vi "Build Flash Command.vi"(8 "error in":errorcluster, 11 "MPLab in":refnum<class "MPLab.lvclass">) -> (0 "error out":errorcluster, 3 "MPLab out":refnum<class "MPLab.lvclass">)   [LabVIEW 2018, in "MPLab.lvlib" / "MPLab.lvclass"]
uses:
  MPLab.lvclass
  Custom Controls/Command Line Options.ctl
  MPLab.lvclass/MPLab.ctl
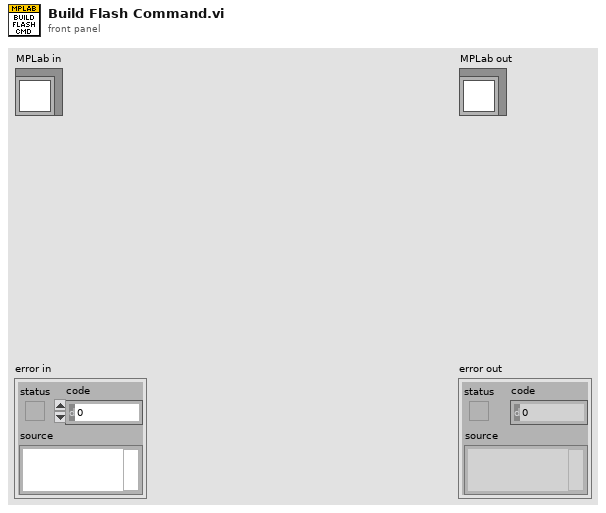
[diagram p1: front panel]
types:
  T1 = typedef "MPLab.lvlib/MPLab.lvclass/Command Line Options.ctl" = enum16{"Blank Check Device", "Erase Flash Device", "Hex File", "Display Device ID", "Display File Checksum", "Low Voltage Programming", "Memory Region", "Part", "Tool", "Verify Device"}
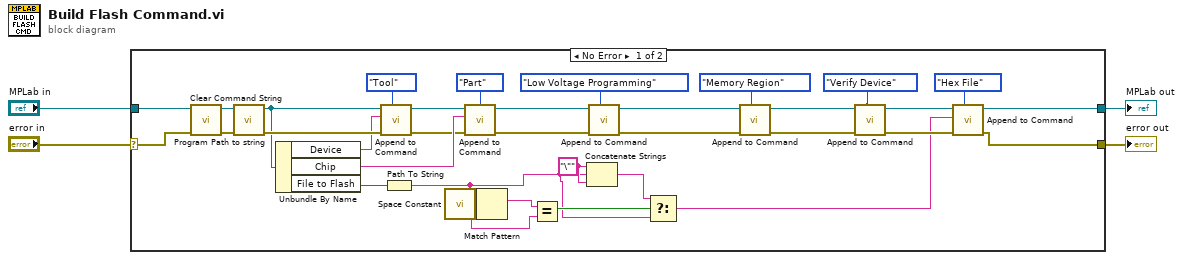
[diagram p0: block diagram]
diagram:
  n1 = case shown="No Error" "error in" {
    selector: "error in" -> [w36 w40]
    tunnel: [w12 w40] -> w3
    tunnel: [w13 w39] -> w1
    tunnel: "MPLab in" -> [w38 w39]
    frame No Error {
      w8 = "\"" ("string")
      n2 = call "Clear Command String.vi"("error in (no error)"=w36, "MPLab in"=w38) -> ("error out"=w35:errorcluster, "MPLab out"=w37:refnum<class "MPLab.lvclass">)  [unwired: 8 in]
      n3 = call "Program Path to string.vi"("error in"=w35, "MPLab in"=w37) -> ("error out"=w34:errorcluster, "MPLab out"=w33:refnum<class "MPLab.lvclass">)  [unwired: 8 in]
      n4 = Unbundle By Name(w33) -> ("Device"=w32:string, "Chip"=w29:string, "File to Flash"=w22:path)
      n5 = call "Append to Command.vi"("Command Line Options"=Command_Line_Options."Tool", "error in (no error)"=w34, "Parameter"=w32, "MPLab in"=w33) -> ("error out"=w23:errorcluster, "MPLab out"=w24:refnum<class "MPLab.lvclass">)  [unwired: 6 in]
      n6 = Path To String(path=w22) -> (string=w6:string)
      n7 = call <vilib>:"Space Constant.vi"() -> ("String"=w10:string)
      n8 = call "Append to Command.vi"("Command Line Options"=Command_Line_Options."Part", "error in (no error)"=w23, "Parameter"=w29, "MPLab in"=w24) -> ("error out"=w20:errorcluster, "MPLab out"=w21:refnum<class "MPLab.lvclass">)  [unwired: 6 in]
      n9 = Match Pattern(string=w6, regular expression=w10) -> (match substring=w11:string)  [unwired: 1 in, 3 out]
      n10 = Equal?(x=w11, y=w10) -> (x = y?=w9:bool)
      n11 = Concatenate Strings(w8, w6, w8) -> (w7:string)
      n12 = call "Append to Command.vi"("Command Line Options"=Command_Line_Options."Low Voltage Programming", "error in (no error)"=w20, "MPLab in"=w21) -> ("error out"=w19:errorcluster, "MPLab out"=w18:refnum<class "MPLab.lvclass">)  [unwired: 7 in]
      n13 = Select(t=w7, s=w9, f=w6) -> (s? t:f=w5:string)
      n14 = call "Append to Command.vi"("Command Line Options"=Command_Line_Options."Memory Region", "error in (no error)"=w19, "MPLab in"=w18) -> ("error out"=w16:errorcluster, "MPLab out"=w17:refnum<class "MPLab.lvclass">)  [unwired: 7 in]
      n15 = call "Append to Command.vi"("Command Line Options"=Command_Line_Options."Verify Device", "error in (no error)"=w16, "MPLab in"=w17) -> ("error out"=w14:errorcluster, "MPLab out"=w15:refnum<class "MPLab.lvclass">)  [unwired: 7 in]
      n16 = call "Append to Command.vi"("Command Line Options"=Command_Line_Options."Hex File", "error in (no error)"=w14, "Parameter"=w5, "MPLab in"=w15) -> ("error out"=w12:errorcluster, "MPLab out"=w13:refnum<class "MPLab.lvclass">)  [unwired: 6 in]
    }
    frame Error {
    }
  }
  "error out" <- w3
  "MPLab out" <- w1
